vi "myxmlparser.vi"() -> ()   [LabVIEW 2011]
doc: "This example demonstrates how to query an XML document by using an XPath expression and returns all the nodes that match the XPath expression."
panel:
  out "output array":T1(array[cluster])
  out "xml_file_content_String":string
  out "Strain_cluster":T2
  out "Voltage_cluster":cluster{dbl, dbl, dbl, dbl, bool, dbl, dbl}
  out "Channel paths":string[](array[string])
  in  "sc":string="/SC0/mod0/ai0/Cluster"
  out "Result Array":string[](array[string])=["<Cluster>\n        <Name/>\n        <NumElts>7</NumElts>\n        <DBL>\n          <Name>max</Name>\n          <Val>10</Val>\n        </DBL>\n        <DBL>\n          <Name>min</Name>\n          <Val>-10</Val>\n        </DBL>\n        <DBL>\n          <Name>factor_a</Name>\n          <Val>22.4</Val>\n        </DBL>\n        <DBL>\n          <Name>factor_b</Name>\n          <Val>0.0</Val>\n        </DBL>\n        <Boolean>\n          <Name>lowpass</Name>\n          <Val>1</Val>\n        </Boolean>\n        <DBL>\n          <Name>lowpassfreq</Name>\n          <Val>60</Val>\n        </DBL>\n        <DBL>\n          <Name>excitation</Name>\n          <Val>10</Val>\n        </DBL>\n      </Cluster>"]
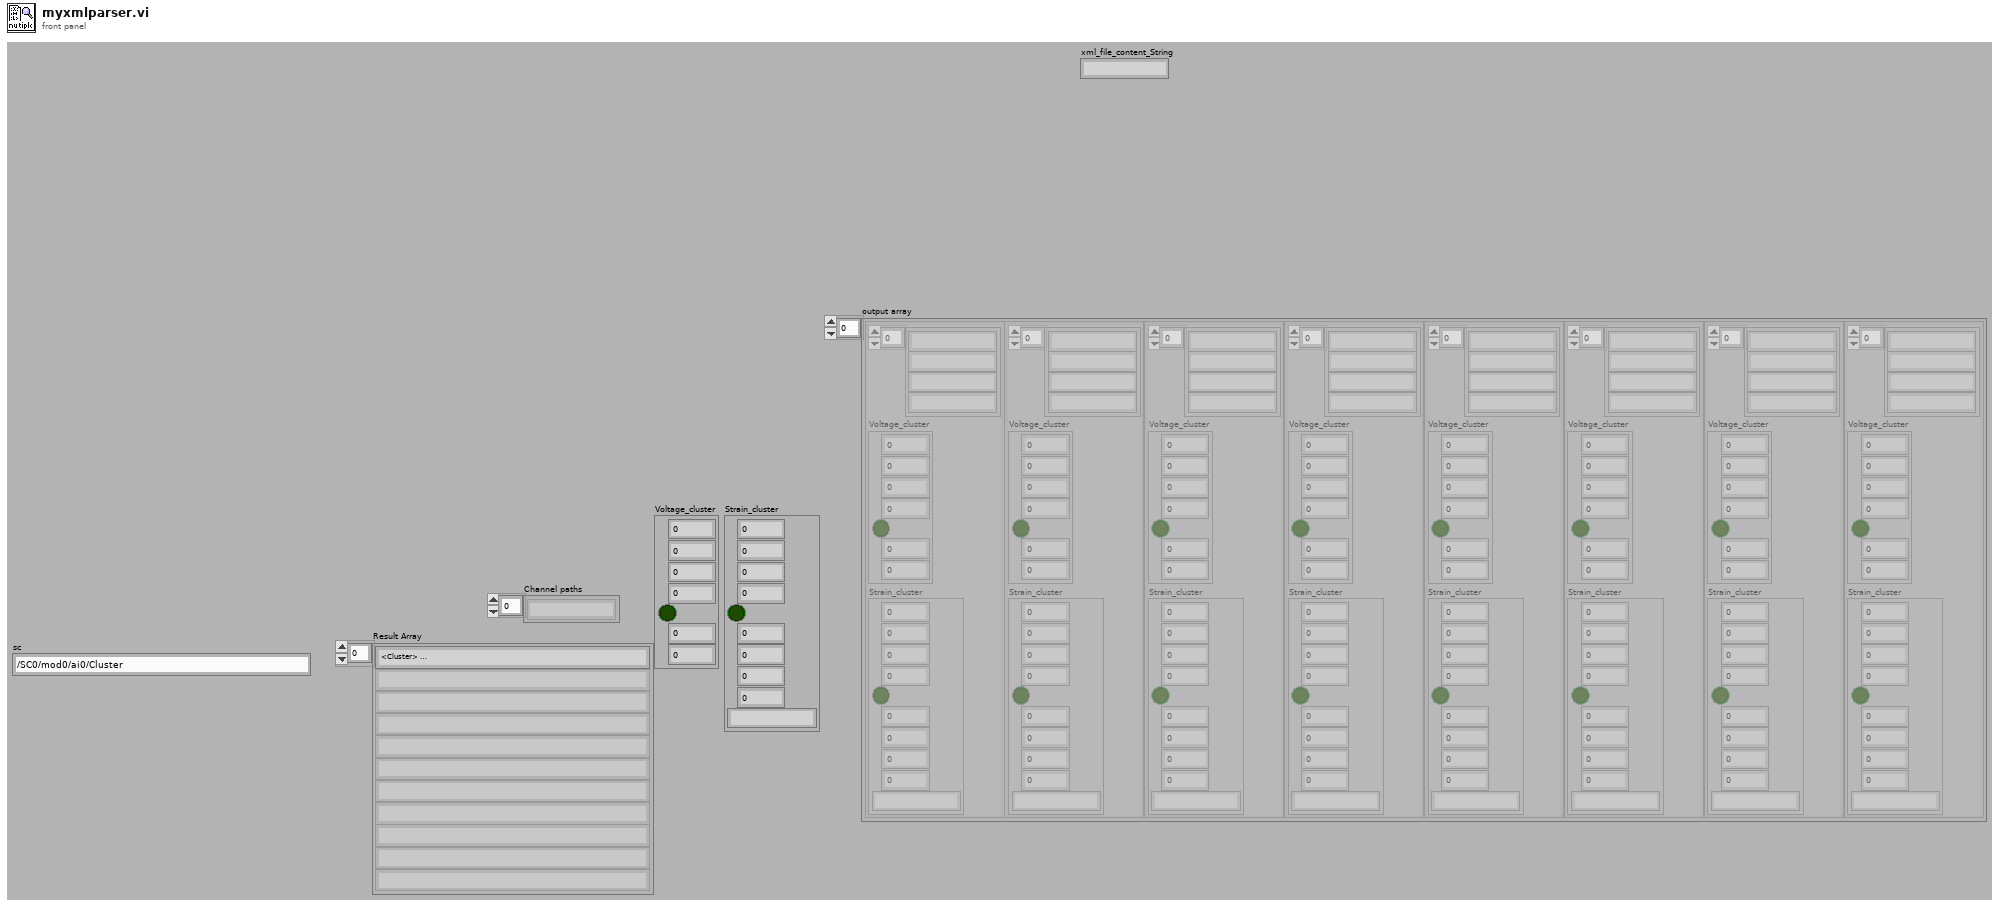
[diagram p1: front panel]
types:
  T1 = cluster{string[], "Voltage_cluster":cluster{dbl, dbl, dbl, dbl, bool, dbl, dbl}, "Strain_cluster":cluster{dbl, dbl, dbl, dbl, bool, dbl, dbl, dbl, dbl, string}}[]
  T2 = cluster{dbl, dbl, dbl, dbl, bool, dbl, dbl, dbl, dbl, string}
  T3 = cluster{string[], "Voltage_cluster":cluster{dbl, dbl, dbl, dbl, bool, dbl, dbl}, "Strain_cluster":cluster{dbl, dbl, dbl, dbl, bool, dbl, dbl, dbl, dbl, string}}
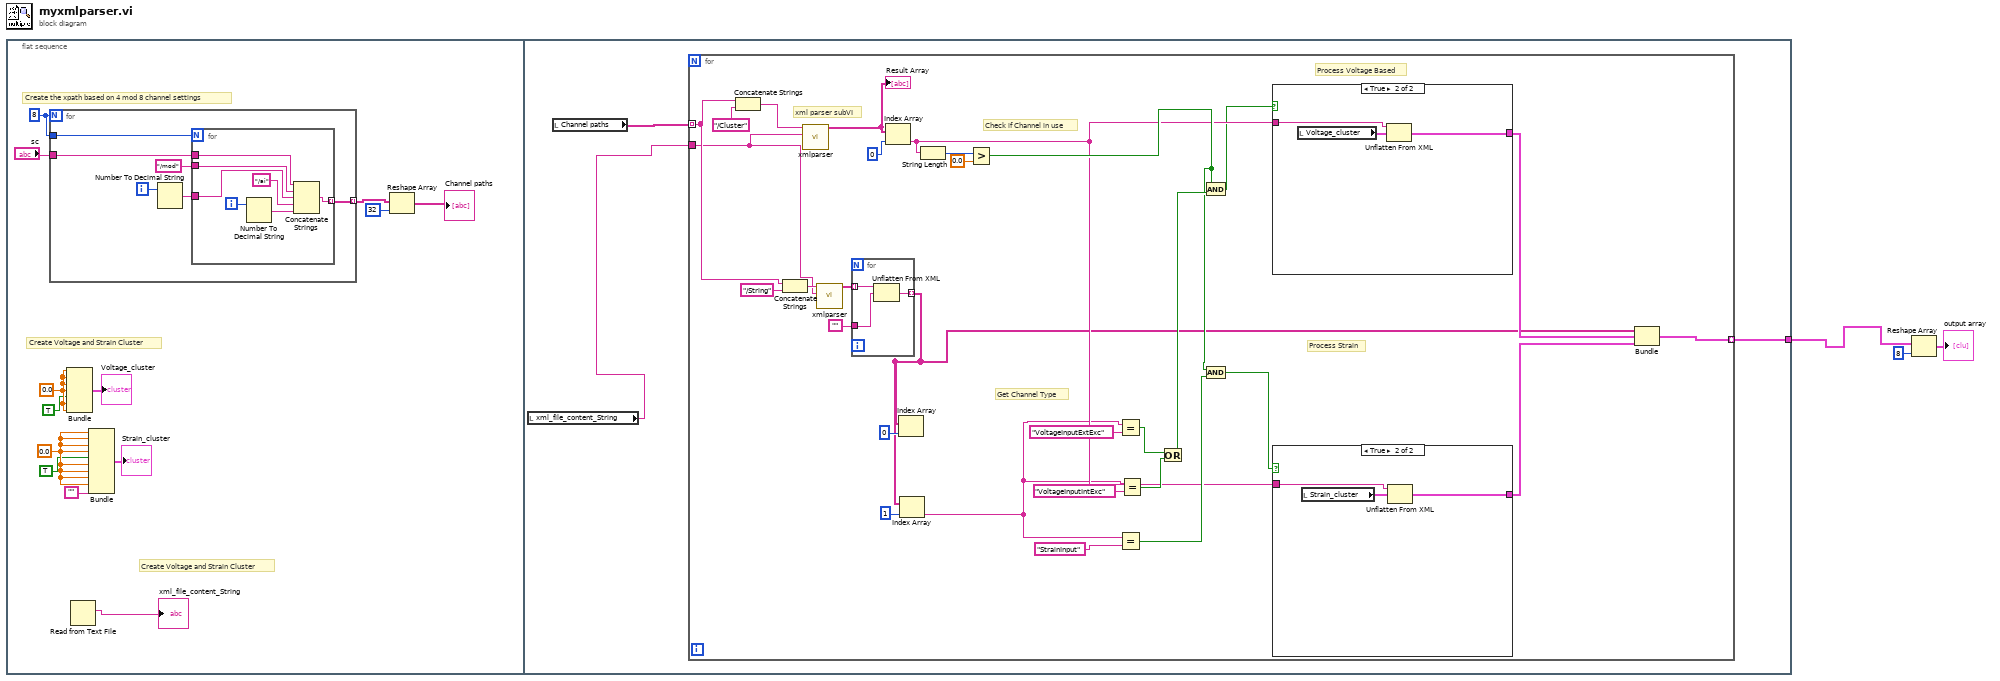
[diagram p0: block diagram]
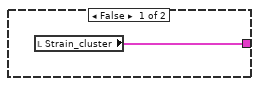
[diagram p2: hidden frame]
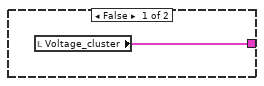
[diagram p3: hidden frame]
diagram:
  n1 = flat-sequence {
    tunnel: [w31] -> w3
    frame #0 {
      w9 = 0.0
      w6 = 0.0
      w15 = 8
      # "Create Voltage and Strain Cluster"
      # "Create Voltage and Strain Cluster"
      # "Create the xpath based on 4 mod 8 channel settings"
      n2 = for {
        N: w15 -> [_]
        tunnel: [w17] -> w14 mode=indexing
        tunnel: "sc" -> [w21]
        tunnel: w15 -> [w18]
        i -> [w22]
        n3 = Number To Decimal String(number=w22) -> (decimal integer string=w19:string)  [unwired: 1 in]
        n4 = for {
          N: w18 -> [_]
          tunnel: w21 -> [w29]
          tunnel: "/mod" -> [w28]
          tunnel: w19 -> [w27]
          tunnel: [w23] -> w17 mode=indexing
          i -> [w25]
          n5 = Number To Decimal String(number=w25) -> (decimal integer string=w24:string)  [unwired: 1 in]
          n6 = Concatenate Strings(w29, w28, w27, "/ai", w24) -> (w23:string)
        }
      }
      n7 = Bundle(w6, w6, w6, w6, TRUE, w6, w6) -> (→"Voltage_cluster":cluster{dbl, dbl, dbl, dbl, bool, dbl, dbl})  [unwired: 1 in]
      n8 = Read from Text File() -> (text=→"xml_file_content_String":string)  [unwired: 4 in, 3 out]
      n9 = Bundle(w9, w9, w9, w9, TRUE, w9, w9, w9, w9, "") -> (→"Strain_cluster":T2)  [unwired: 1 in]
      n10 = Reshape Array(w14, 32 ("dimension size")) -> (→"Channel paths":string[])
    }
    frame #1 {
      n11 = local read "xml_file_content_String"() -> (w30:string)
      n12 = local read "Channel paths"() -> (w32:string[])
      n13 = for {
        tunnel: w30 -> [w53]
        tunnel: w32 -> [w54] mode=indexing
        tunnel: [w34] -> w31 mode=indexing
        # "Process Strain"
        # "Process Voltage Based"
        # "Check if Channel in use"
        # "Get Channel Type"
        # "xml parser subVI"
        n14 = Concatenate Strings(w54, "/Cluster") -> (w57:string)
        n15 = Concatenate Strings(w54, "/String") -> (w55:string)
        n16 = call "xmlparser.vi"("xml_file_content"=w53, "XPath expression"=w57) -> ("Array 2"=w59:string[])  [unwired: 9 in]
        "Result Array" <- w59
        n17 = call "xmlparser.vi"("xml_file_content"=w53, "XPath expression"=w55) -> ("Array 2"=w41:string[])  [unwired: 9 in]
        n18 = for {
          tunnel: w41 -> [w65] mode=indexing
          tunnel: "" -> [w64]
          tunnel: [w63] -> w33 mode=indexing
          n19 = Unflatten From XML(xml string=w65, type=w64) -> (value=w63:string)  [unwired: 1 in, 1 out]
        }
        n20 = Index Array(array=w59, index=0) -> (element=w43:string)
        n21 = Index Array(array=w33, index=0) -> ()  [unwired: 1 out]
        n22 = Index Array(array=w33, index=1) -> (element=w37:string)
        n23 = String Length(string=w43) -> (length=w62:i32)
        n24 = Greater?(x=w62, y=0.0) -> (0:w46:bool)
        n25 = Equal?(x=w37, y="VoltageInputExtExc") -> (x = y?=w50:bool)
        n26 = Equal?(x=w37, y="StrainInput") -> (x = y?=w45:bool)
        n27 = Equal?(x=w37, y="VoltageInputIntExc") -> (x = y?=w49:bool)
        n28 = Or(x=w50, y=w49) -> (x .or. y?=w48:bool)
        n29 = And(x=w46, y=w48) -> (x .and. y?=w42:bool)
        n30 = And(x=w46, y=w45) -> (x .and. y?=w44:bool)
        n31 = case shown="True" w42 {
          tunnel: w43 -> [_ w73]
          tunnel: [w70 w72] -> w36
          frame False {
            n32 = local read "Voltage_cluster"() -> (w70:cluster{dbl, dbl, dbl, dbl, bool, dbl, dbl})
          }
          frame True {
            n33 = local read "Voltage_cluster"() -> (w71:cluster{dbl, dbl, dbl, dbl, bool, dbl, dbl})
            n34 = Unflatten From XML(xml string=w73, type=w71) -> (value=w72:cluster{dbl, dbl, dbl, dbl, bool, dbl, dbl})  [unwired: 1 in, 1 out]
          }
        }
        n35 = case shown="True" w44 {
          tunnel: w43 -> [_ w69]
          tunnel: [w66 w68] -> w35
          frame False {
            n36 = local read "Strain_cluster"() -> (w66:T2)
          }
          frame True {
            n37 = local read "Strain_cluster"() -> (w67:T2)
            n38 = Unflatten From XML(xml string=w69, type=w67) -> (value=w68:T2)  [unwired: 1 in, 1 out]
          }
        }
        n39 = Bundle(w33, "Voltage_cluster"=w36, "Strain_cluster"=w35) -> (w34:T3)  [unwired: 1 in]
      }
    }
  }
  n40 = Reshape Array(w3, 8 ("dimension size")) -> (→"output array":T1)
